vi "Actor Core.vi"(8 "error in":errorcluster, 11 "IViewModel In":refnum<class "IViewModel.lvclass">) -> (0 "error out":errorcluster, 3 "Actor out":refnum<class "Actor.lvclass">)   [LabVIEW 2017, in "IViewModel.lvlib" / "IViewModel.lvclass"]
doc: "(<B>Filename</B>: Actor Framework.lvlib:Actor.lvclass:Actor Core.vi)\n\nReceives messages to the actor, reacts to them, and initiates any error handling that may shut the actor down.\n\nDescendant classes may override this VI to append parallel tasks for the actor to complete while it handles messages. Overrides use the Call Parent Method node.\n\n<License>\nCopyright © 2017 Composed Systems, LLC | All rights reserved\nwww.composed.io\n\nAuthor: Ethan Stern <ethan.stern@composed.io>\n\nThis software is provided \"AS IS\" WITHOUT WARRANTIES, either express or implied, AND IS FOR EDUCATIONAL PURPOSES ONLY.\n</License>"
uses:
  IViewModel.lvclass
  C:/Git/mva-framework/Source/Framework/ActorEvents/IEventAggregator/IEventAggregator.lvclass
  <vilib>/ActorFramework/Actor/Actor.lvclass
  <vilib>/event_ctls.llb/lveventtype.ctl
  IViewModel.lvclass/IViewModel.ctl
  IViewable/ProtectedSubpanel/Release Protected Subpanel.vi
  IViewManager/IViewManager/IViewManager.lvclass
  ActorEvents/IEventAggregator/IEventAggregator.lvclass
  IViewable/ProtectedSubpanel/ProtectedSubpanel.lvclass
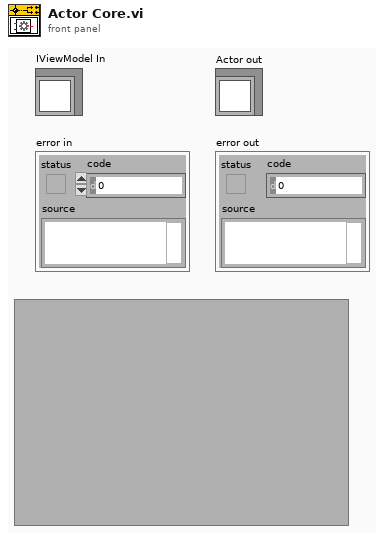
[diagram p1: front panel]
types:
  T1 = typedef "lveventtype.ctl" = enum32{"Null", "Timeout", "Annotation Menu Selection", "Annotation Menu Selection?", "App Instance Close", "App Instance Close?", "Autoscale Range Change", "Bookmark Info Change", "Cell Edit", "Cell Edit?", "Cursor Grab", "Cursor Grab?", "Cursor Menu Selection", "Cursor Menu Selection?", "Cursor Move", "Cursor Release", "Data Change", "Direction Change", "Display State Change", "Drag Ended", "Drag Enter", "Drag Leave", "Drag Over", "Drag Source Update", "Drag Starting", "Drag Starting?", "Drop", "Exec State Change", "Key Down", "Key Down?", "Key Repeat", "Key Repeat?", "Key Up", "Listbox Double Click", "Menu Activation?", "Menu Selection (App)", "Menu Selection? (App)", "Menu Selection (User)", "Mouse Down", "Mouse Down?", "Mouse Enter", "Mouse Leave", "Mouse Move", "Mouse Up", "Mouse Wheel", "NI Security User Change (App)", "Pane Size", "Panel Close", "Panel Close?", "Panel Resize", "Plot Attribute Change", "Scale Range Change", "Shortcut Menu Activation?", "Shortcut Menu Selection (App)", "Shortcut Menu Selection? (App)", "Shortcut Menu Selection (User)", "Tree Double Click", "Tree Drag", "Tree Drag?", "Tree Drop", "Tree Drop?", "Tree Item Close", "Tree Item Close?", "Tree Item Open", "Tree Item Open?", "User Event", "Value Change"}
  T2 = typedef "IViewable.lvlib/ProtectedSubpanel.lvclass/Protected Subpanel Reference.ctl" = refnum<data-value>
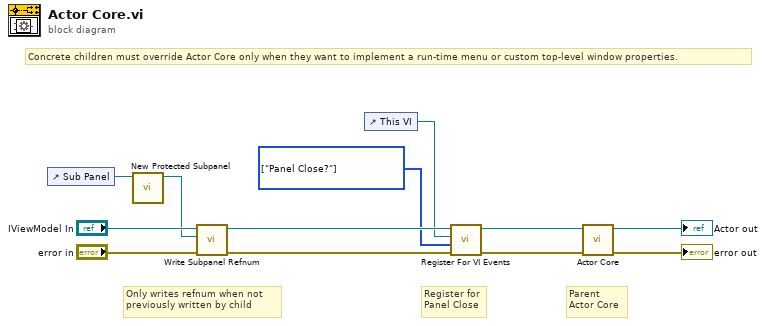
[diagram p0: block diagram]
diagram:
  w3 = T1[] [enum."Panel Close?"] items=["Null", "Timeout", "Annotation Menu Selection", "Annotation Menu Selection?", "App Instance Close", "App Instance Close?", "Autoscale Range Change", "Bookmark Info Change", "Cell Edit", "Cell Edit?", "Cursor Grab", "Cursor Grab?", "Cursor Menu Selection", "Cursor Menu Selection?", "Cursor Move", "Cursor Release", "Data Change", "Direction Change", "Display State Change", "Drag Ended", "Drag Enter", "Drag Leave", "Drag Over", "Drag Source Update", "Drag Starting", "Drag Starting?", "Drop", "Exec State Change", "Key Down", "Key Down?", "Key Repeat", "Key Repeat?", "Key Up", "Listbox Double Click", "Menu Activation?", "Menu Selection (App)", "Menu Selection? (App)", "Menu Selection (User)", "Mouse Down", "Mouse Down?", "Mouse Enter", "Mouse Leave", "Mouse Move", "Mouse Up", "Mouse Wheel", "NI Security User Change (App)", "Pane Size", "Panel Close", "Panel Close?", "Panel Resize", "Plot Attribute Change", "Scale Range Change", "Shortcut Menu Activation?", "Shortcut Menu Selection (App)", "Shortcut Menu Selection? (App)", "Shortcut Menu Selection (User)", "Tree Double Click", "Tree Drag", "Tree Drag?", "Tree Drop", "Tree Drop?", "Tree Item Close", "Tree Item Close?", "Tree Item Open", "Tree Item Open?", "User Event", "Value Change"] ("Registration Types")
  # "Parent\nActor Core"
  # "Register for\nPanel Close"
  # "Only writes refnum when not\npreviously written by child"
  # "Concrete children must override Actor Core only when they want to implement a run-time menu or custom top-level window properties."
  n1 = control-ref of="Sub Panel"() -> (w2:refnum<vi>)
  n2 = call "New Protected Subpanel.vi"("SubPnl Refnum"=w2) -> ("Protected Subpanel"=w1:T2)  [unwired: 9 in, 1 out]
  n3 = call "Write Subpanel Refnum.vi"("error in (no error)"="error in", "Protected Subpanel"=w1, "IViewModel In"="IViewModel In") -> ("error out"=w6:errorcluster, "IViewModel Out"=w11:refnum<class "IViewModel.lvclass">)  [unwired: 7 in]
  n4 = control-ref of="This VI"() -> (w4:refnum<vi>)
  n5 = call "Register For VI Events.vi"("error in (no error)"=w6, "Registration Types"=w3, "VI Refnum"=w4, "IEventAggregator In"=w11) -> ("error out"=w5:errorcluster, "IEventAggregator Out"=w7:refnum<class "IViewModel.lvclass">)  [unwired: 6 in]
  n6 = call-parent "Actor Core.vi"("error in"=w5, "IViewable In"=w7) -> ("error out"=→"error out":errorcluster, "Actor out"=→"Actor out":refnum<class "Actor.lvclass">)  [unwired: 8 in]
